vi "Find_USB.vi"(9 "USB索引":u8) -> (0 "错误输出":errorcluster, 2 "元素":string)   [LabVIEW 2014]
panel:
  out "返回数":u32
  out "查找列表":string[](array[string])
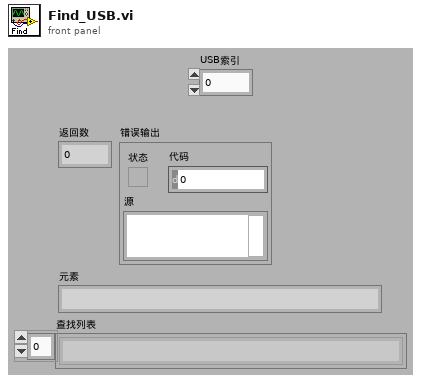
[diagram p1: front panel]
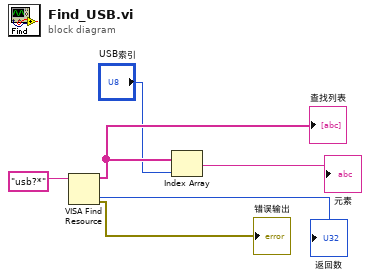
[diagram p0: block diagram]
diagram:
  n1 = VISA Find Resource(11:"usb?*" ("表达式(\"?*\")")) -> (0:→"错误输出":errorcluster, 2:→"返回数":u32, 3:w3:string[])  [unwired: 2 in]
  "查找列表" <- w3
  n2 = Index Array(array=w3, index="USB索引") -> (element=→"元素":string)
